vi "Write Fine regions' centers mask.vi"(8 "error in (no error)":errorcluster, 10 "Fine regions' centers mask":dbl[](array[numeric]), 11 "Update Focus Msg in":refnum<class "Update Focus Msg.lvclass">) -> (0 "error out":errorcluster, 3 "Update Focus Msg out":refnum<class "Update Focus Msg.lvclass">)   [LabVIEW 2016, in "Update Focus Msg.lvclass"]
uses:
  Update Focus Msg.lvclass
  Update Focus Msg.lvclass/Update Focus Msg.ctl
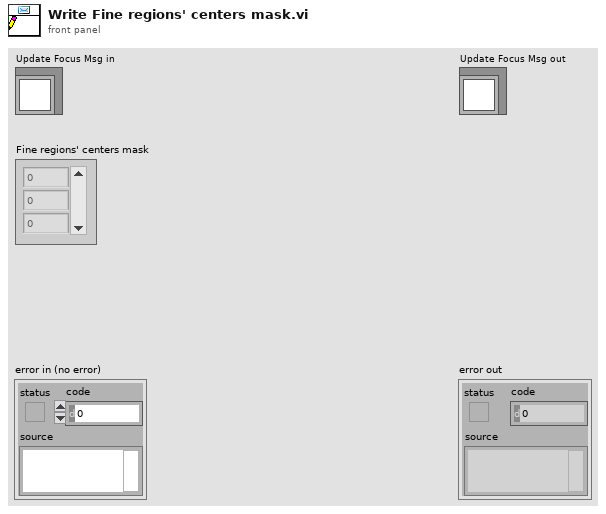
[diagram p1: front panel]
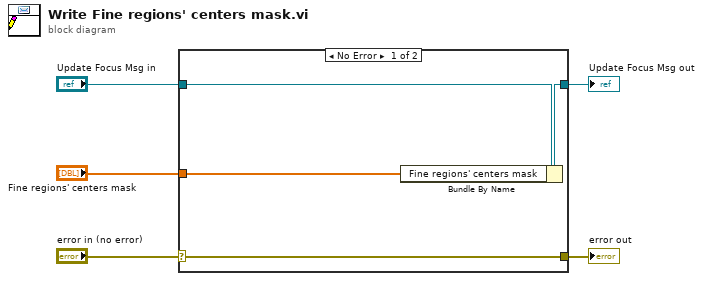
[diagram p0: block diagram]
diagram:
  n1 = case shown="No Error" "error in (no error)" {
    selector: "error in (no error)" -> [w9 w10]
    tunnel: [w9 w10] -> w4
    tunnel: [w7 w11] -> w2
    tunnel: "Update Focus Msg in" -> [w8 w11]
    tunnel: "Fine regions' centers mask" -> [w6 _]
    frame No Error {
      n2 = Bundle By Name(cluster=w8, "Fine regions' centers mask"=w6) -> (w7:refnum<class "Update Focus Msg.lvclass">)
    }
    frame Error {
    }
  }
  "error out" <- w4
  "Update Focus Msg out" <- w2
